vi "Handle PUBLISHED.vi"(8 "error in (no error)":errorcluster, 9 "Message Loop data (in)":T1, 10 "WAMP Message":T14 {"Message Codes" items=["HELLO"=1, "WELCOME"=2, "ABORT"=3, "GOODBYE"=6, "ERROR"=8, "PUBLISH"=16, "PUBLISHED"=17, "SUBSCRIBE"=32, "SUBSCRIBED"=33, "UNSUBSCRIBE"=34, "UNSUBSCRIBED"=35, "EVENT"=36, "CALL"=48, "RESULT"=59, "REGISTER"=64, "REGISTERED"=65, "UNREGISTER"=66, "UNREGISTERED"=67, "INVOCATION"=68, "YIELD"=70]}, 11 "reference":refnum<class "WAMP Client.lvclass">) -> (0 "error out":errorcluster, 1 "Message Loop data (out)":T1, 3 "reference out":refnum<class "WAMP Client.lvclass">)   [LabVIEW 2020, in "wamplv.lvlib" / "WAMP Client.lvclass"]
uses:
  <vilib>/samangh/wamplv/WAMP Client/WAMP Client.lvclass
  <vilib>/samangh/wamplv/WAMP Client/WAMP Client.lvclass/WAMP Client.ctl
  <vilib>/samangh/wamplv/WAMP Client/TypeDef/PUBLISH Result.ctl
  <vilib>/samangh/wamplv/WAMP Client/TypeDef/WAMP Error Payload.ctl
  <vilib>/samangh/wamplv/WAMP Client/TypeDef/Combined error.ctl
  <vilib>/samangh/wamplv/WAMP Message Codes.ctl
  <vilib>/samangh/wamplv/WAMP Client/TypeDef/WAMP Received Message.ctl
  <vilib>/samangh/wamplv/WAMP Client/TypeDef/PUBLISH Request Data.ctl
  <vilib>/samangh/wamplv/WAMP Client/TypeDef/Publish Requests Map.ctl
  <vilib>/samangh/wamplv/WAMP Client/TypeDef/REGISTERED or ERROR payload.ctl
  <vilib>/samangh/wamplv/WAMP Client/TypeDef/INVOCATION payload.ctl
  <vilib>/samangh/wamplv/WAMP Client/TypeDef/REGISTER Request Data.ctl
  <vilib>/samangh/wamplv/WAMP Client/TypeDef/Endpoint Data.ctl
  <vilib>/samangh/wamplv/WAMP Client/TypeDef/RESULT Payload.ctl
  <vilib>/samangh/wamplv/WAMP Client/TypeDef/CALL Request Data.ctl
  <vilib>/samangh/wamplv/WAMP Client/TypeDef/CALL Request Map.ctl
  <vilib>/samangh/wamplv/WAMP Client/TypeDef/Event Payload.ctl
  <vilib>/samangh/wamplv/WAMP Client/TypeDef/Subscribe Result.ctl
  <vilib>/samangh/wamplv/WAMP Client/TypeDef/SUBSCRIBE Request Data.ctl
  <vilib>/samangh/wamplv/WAMP Client/TypeDef/SUBSCRIBE Requests Map.ctl
  <vilib>/samangh/wamplv/WAMP Client/TypeDef/Subscription Details.ctl
  <vilib>/samangh/wamplv/WAMP Client/TypeDef/Subscriptions Map.ctl
  <vilib>/samangh/wamplv/WAMP Client/TypeDef/UNSUBSCRIBE Result.ctl
  <vilib>/samangh/wamplv/WAMP Client/TypeDef/UNSUBSCRIBE Request Data.ctl
  <vilib>/samangh/wamplv/WAMP Client/TypeDef/Unsubscribe Requests Map.ctl
  <vilib>/samangh/wamplv/WAMP Client/TypeDef/Message Loop Shift Reg Data.ctl
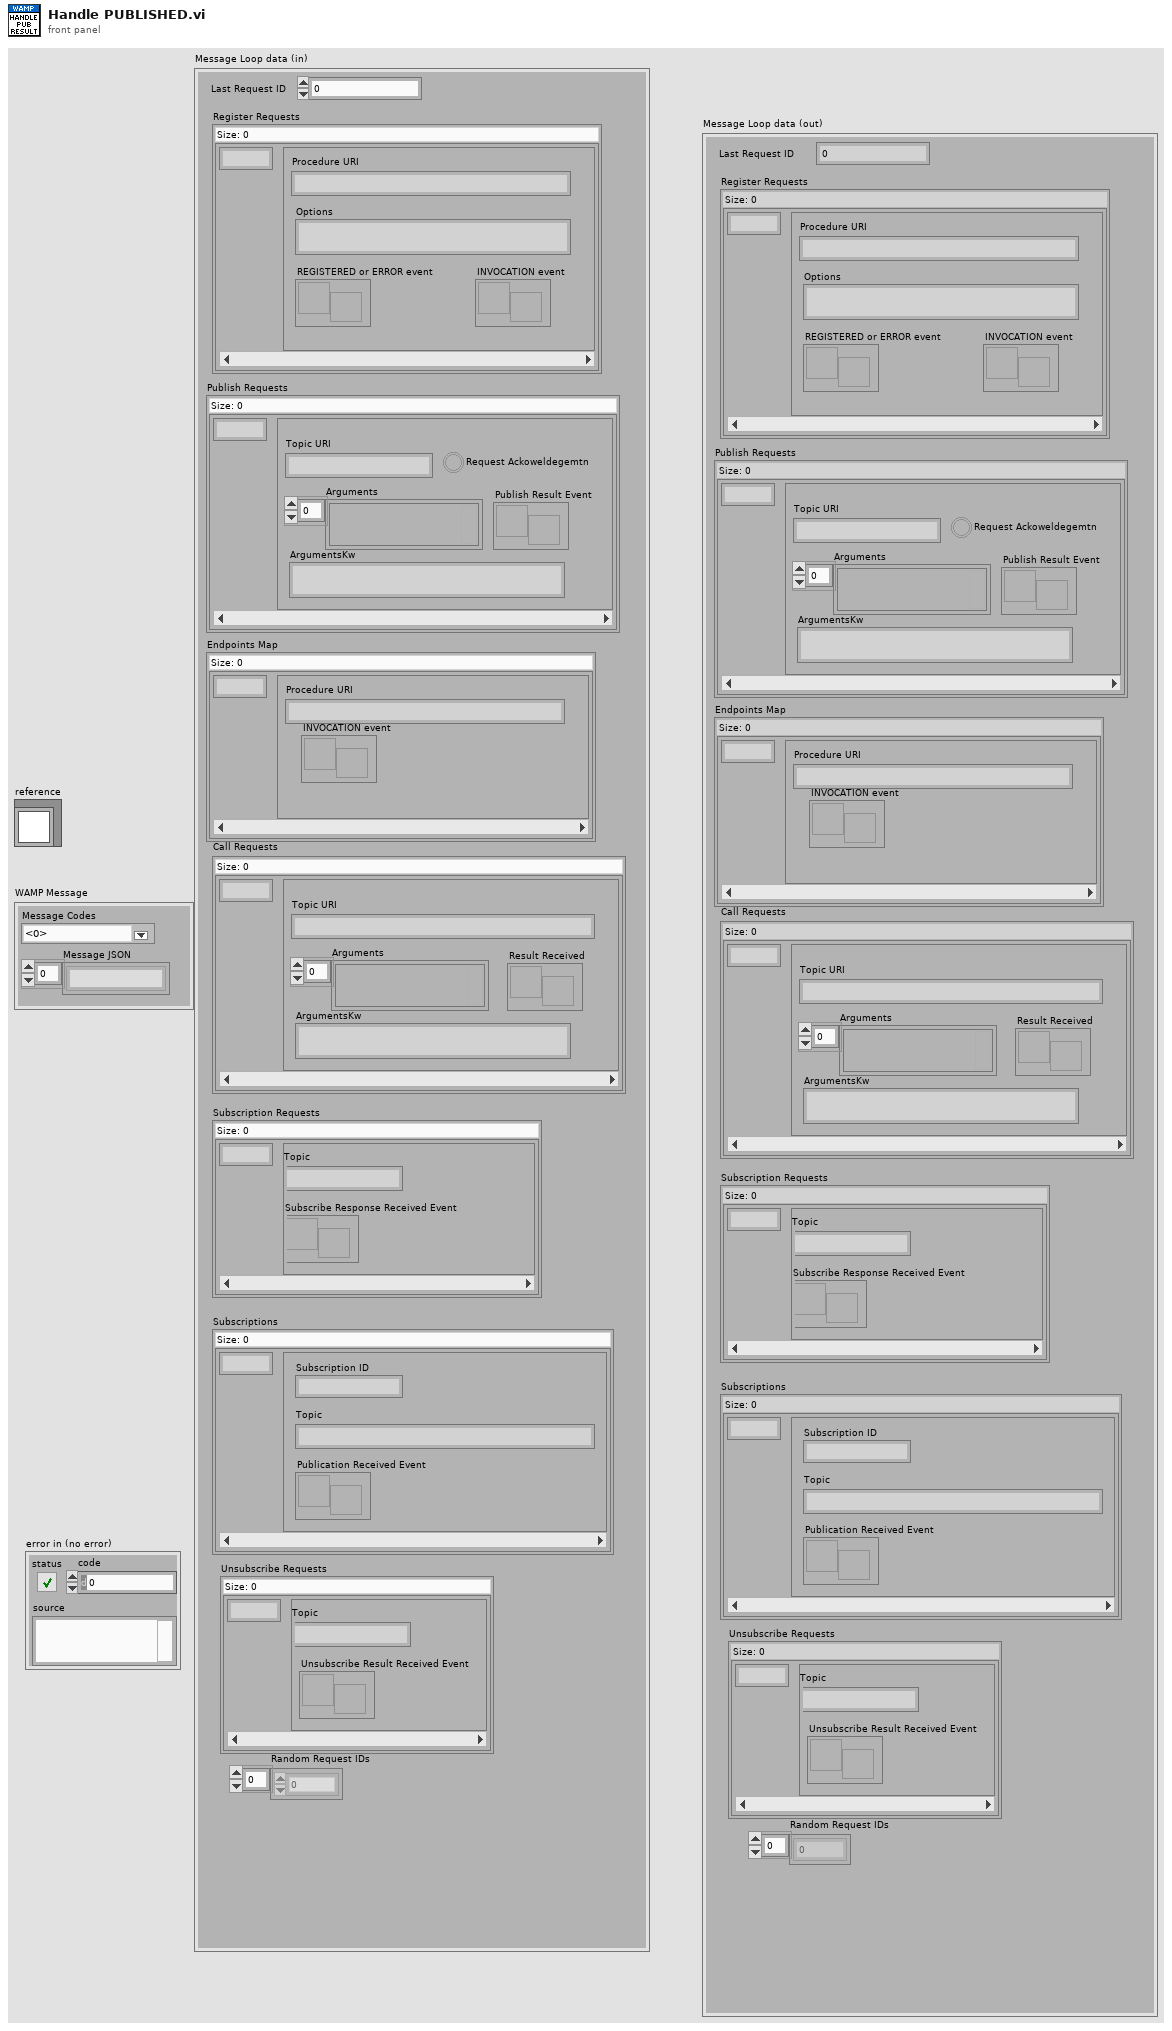
[diagram p1: front panel]
types:
  T1 = typedef "wamplv.lvlib/WAMP Client.lvclass/Message Loop Shift Reg Data.ctl" = cluster{"Last Request ID":u64, "Register Requests":map{u64, T2}, "Publish Requests":T3, "Endpoints Map":map{u64, T5}, "Call Requests":T6, "Subscription Requests":T8, "Subscriptions":T10, "Unsubscribe Requests":T12, "Random Request IDs":u64[]}
  T2 = typedef "wamplv.lvlib/WAMP Client.lvclass/REGISTER Request Data.ctl" = cluster{"Procedure URI":string, "Options":string, "REGISTERED or ERROR event":refnum<user-event>, "INVOCATION event":refnum<user-event>}
  T3 = typedef "wamplv.lvlib/WAMP Client.lvclass/Publish Requests Map.ctl" = map{u64, T4}
  T4 = typedef "wamplv.lvlib/WAMP Client.lvclass/PUBLISH Request Data.ctl" = cluster{"Topic URI":string, "Arguments":variant[], "ArgumentsKw":string, "Publish Result Event":refnum<user-event>, "Request Ackoweldegemtn":bool}
  T5 = typedef "wamplv.lvlib/WAMP Client.lvclass/Endpoint Data.ctl" = cluster{"Procedure URI":string, "INVOCATION event":refnum<user-event>}
  T6 = typedef "wamplv.lvlib/WAMP Client.lvclass/CALL Request Map.ctl" = map{u64, T7}
  T7 = typedef "wamplv.lvlib/WAMP Client.lvclass/CALL Request Data.ctl" = cluster{"Topic URI":string, "Arguments":variant[], "ArgumentsKw":string, "Result Received":refnum<user-event>}
  T8 = typedef "wamplv.lvlib/WAMP Client.lvclass/SUBSCRIBE Requests Map.ctl" = map{u64, T9}
  T9 = typedef "wamplv.lvlib/WAMP Client.lvclass/SUBSCRIBE Request Data.ctl" = cluster{"Topic":string, "Subscribe Response Received Event":refnum<user-event>}
  T10 = typedef "wamplv.lvlib/WAMP Client.lvclass/Subscriptions Map.ctl" = map{u64, T11}
  T11 = typedef "wamplv.lvlib/WAMP Client.lvclass/Subscription Details.ctl" = cluster{"Subscription ID":u64, "Topic":string, "Publication Received Event":refnum<user-event>}
  T12 = typedef "wamplv.lvlib/WAMP Client.lvclass/Unsubscribe Requests Map.ctl" = map{u64, T13}
  T13 = typedef "wamplv.lvlib/WAMP Client.lvclass/UNSUBSCRIBE Request Data.ctl" = cluster{"Topic":string, "Unsubscribe Result Received Event":refnum<user-event>}
  T14 = typedef "wamplv.lvlib/WAMP Client.lvclass/WAMP Received Message.ctl" = cluster{"Message JSON":string[], "Message Codes":T15}
  T15 = typedef "wamplv.lvlib/WAMP Client.lvclass/WAMP Message Codes.ctl" = u16
  T16 = typedef "wamplv.lvlib/WAMP Client.lvclass/PUBLISH Result.ctl" = cluster{"Publish Request ID":u64, "Publication ID":u64, "Success?":bool, "Combined Error":T17}
  T17 = typedef "wamplv.lvlib/WAMP Client.lvclass/Combined error.ctl" = cluster{"Error?":bool, "WAMP Error":T18, "Error":errorcluster}
  T18 = typedef "wamplv.lvlib/WAMP Client.lvclass/WAMP Error Payload.ctl" = cluster{"Details":string, "ArgumentKw Payload":string, "Wamp error?":bool, "Error URI":string, "Arguments Payload":string[]}
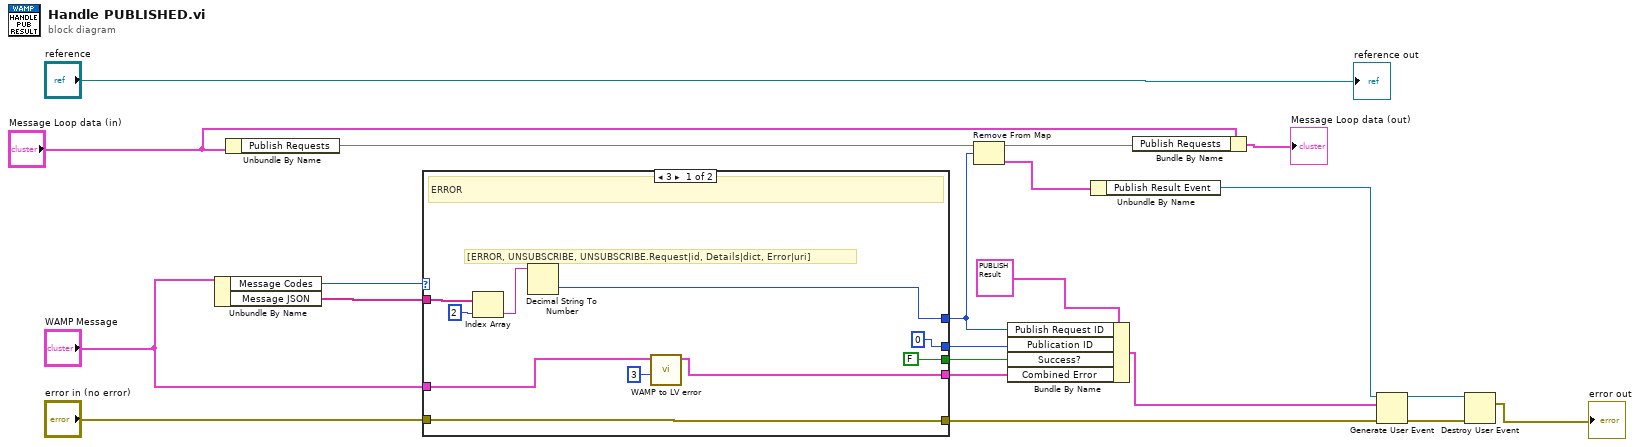
[diagram p0: block diagram]
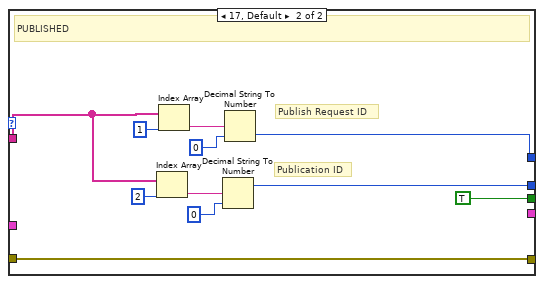
[diagram p2: hidden frame]
diagram:
  n1 = Unbundle By Name("WAMP Message") -> ("Message Codes"=w16:T15, "Message JSON"=w15:string[])
  n2 = Unbundle By Name("Message Loop data (in)") -> ("Publish Requests"=w6:T3)
  n3 = case shown="3" w16 {
    tunnel: w15 -> [w29 w33]
    tunnel: [w26 w37] -> w9
    tunnel: "error in (no error)" -> [w28 w41]
    tunnel: [w28 w41] -> w18
    tunnel: [FALSE ("Success?") TRUE ("Success?")] -> w20
    tunnel: [0 ("offset past number") w32] -> w8
    tunnel: "WAMP Message" -> [w24 _]
    tunnel: [w22 _] -> w1
    frame 3 {
      # "[ERROR, UNSUBSCRIBE, UNSUBSCRIBE.Request|id, Details|dict, Error|uri]"
      # "ERROR"
      n4 = Index Array(array=w29, index=2) -> (element=w30:string)
      n5 = Decimal String To Number(string=w30) -> (number=w26:i32)  [unwired: 2 in, 1 out]
      n6 = call <vilib>:"WAMP to LV error.vi"("Details Index"=u32 3, "WAMP Message"=w24) -> ("Combined Error"=w22:T17)  [unwired: 7 in, 2 out]
    }
    frame 17, Default {
      # "Publication ID"
      # "Publish Request ID"
      # "PUBLISHED"
      n7 = Index Array(array=w33, index=2) -> (element=w35:string)
      n8 = Index Array(array=w33, index=1) -> (element=w39:string)
      n9 = Decimal String To Number(string=w35, default (0L)=u64 0) -> (offset past number=w32:i32)  [unwired: 1 in, 1 out]
      n10 = Decimal String To Number(string=w39, default (0L)=u64 0) -> (number=w37:u64)  [unwired: 1 in, 1 out]
    }
  }
  n11 = Remove From Map(10:w9, 11:w6) -> (1:w14:T4, 3:w5:T3)  [unwired: 1 out]
  n12 = Bundle By Name(cluster=T16 {"Publish Request ID"=0, "Publication ID"=0, "Success?"=FALSE, "Combined Error"={"Error?"=FALSE, "WAMP Error"={"Details"="", "ArgumentKw Payload"="{}", "Wamp error?"=FALSE, "Error URI"="", "Arguments Payload"=[]}, "Error"={"status"=FALSE, "code"=0, "source"=""}}} ("Cluster"), "Publish Request ID"=w9, "Publication ID"=w8, "Success?"=w20, "Combined Error"=w1) -> (w19:T16)
  n13 = Unbundle By Name(w14) -> ("Publish Result Event"=w7:refnum<user-event>)
  n14 = Bundle By Name(cluster="Message Loop data (in)", "Publish Requests"=w5) -> (→"Message Loop data (out)":T1)
  n15 = Generate User Event(user event=w7, event data cluster=w19, error in=w18) -> (user event out=w11:refnum<user-event>, error out=w13:errorcluster)  [unwired: 1 in]
  n16 = Destroy User Event(user event=w11, error in=w13) -> (error out=→"error out":errorcluster)
  "reference out" <- "reference"
